vi "createTelemetry.vi"(8 "error in (no error)":errorcluster, 11 "UserEvents in":refnum<class "UserEvents.lvclass">) -> (0 "error out":errorcluster, 3 "UserEvents out":refnum<class "UserEvents.lvclass">)   [LabVIEW 2016, in "UserEvents.lvclass"]
uses:
  UserEvents.lvclass
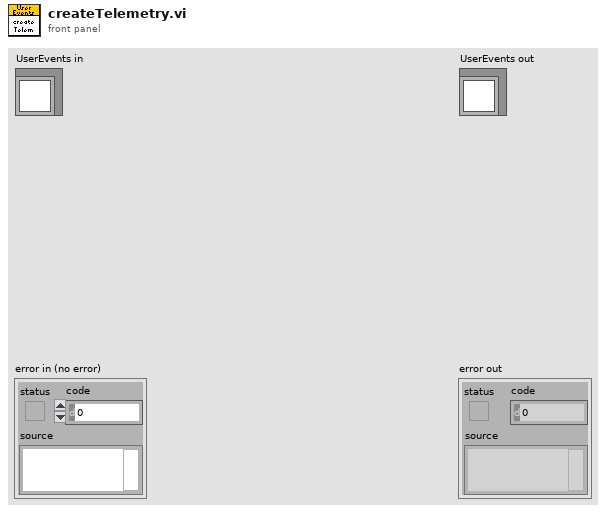
[diagram p1: front panel]
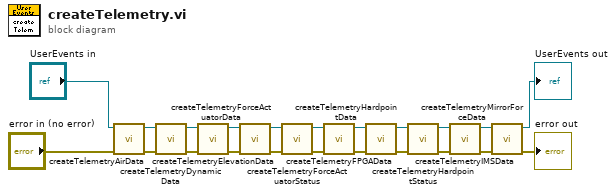
[diagram p0: block diagram]
diagram:
  n1 = call "createTelemetryAirData.vi"("error in (no error)"="error in (no error)", "UserEvents in"="UserEvents in") -> ("error out"=w10:errorcluster, "UserEvents out"=w21:refnum<class "UserEvents.lvclass">)  [unwired: 8 in]
  n2 = call "createTelemetryDynamicData.vi"("error in (no error)"=w10, "UserEvents in"=w21) -> ("error out"=w9:errorcluster, "UserEvents out"=w20:refnum<class "UserEvents.lvclass">)  [unwired: 8 in]
  n3 = call "createTelemetryElevationData.vi"("error in (no error)"=w9, "UserEvents in"=w20) -> ("error out"=w8:errorcluster, "UserEvents out"=w19:refnum<class "UserEvents.lvclass">)  [unwired: 8 in]
  n4 = call "createTelemetryForceActuatorData.vi"("error in (no error)"=w8, "UserEvents in"=w19) -> ("error out"=w7:errorcluster, "UserEvents out"=w18:refnum<class "UserEvents.lvclass">)  [unwired: 8 in]
  n5 = call "createTelemetryForceActuatorStatus.vi"("error in (no error)"=w7, "UserEvents in"=w18) -> ("error out"=w6:errorcluster, "UserEvents out"=w17:refnum<class "UserEvents.lvclass">)  [unwired: 8 in]
  n6 = call "createTelemetryFPGAData.vi"("error in (no error)"=w6, "UserEvents in"=w17) -> ("error out"=w5:errorcluster, "UserEvents out"=w16:refnum<class "UserEvents.lvclass">)  [unwired: 8 in]
  n7 = call "createTelemetryHardpointData.vi"("error in (no error)"=w5, "UserEvents in"=w16) -> ("error out"=w4:errorcluster, "UserEvents out"=w15:refnum<class "UserEvents.lvclass">)  [unwired: 8 in]
  n8 = call "createTelemetryHardpointStatus.vi"("error in (no error)"=w4, "UserEvents in"=w15) -> ("error out"=w3:errorcluster, "UserEvents out"=w14:refnum<class "UserEvents.lvclass">)  [unwired: 8 in]
  n9 = call "createTelemetryIMSData.vi"("error in (no error)"=w3, "UserEvents in"=w14) -> ("error out"=w2:errorcluster, "UserEvents out"=w13:refnum<class "UserEvents.lvclass">)  [unwired: 8 in]
  n10 = call "createTelemetryMirrorForceData.vi"("error in (no error)"=w2, "UserEvents in"=w13) -> ("error out"=→"error out":errorcluster, "UserEvents out"=→"UserEvents out":refnum<class "UserEvents.lvclass">)  [unwired: 8 in]
